vi "ButtonEvents.vi"(11 "UiDefinition":T1) -> ()   [LabVIEW 2020]
uses:
  UIReferences.ctl
  C:/Users/User/Desktop/Automation/NextVersion2/LabviewDXFViewer/bin/Release/LabviewDXFViewer.exe
  LabviewDXFViewer/bin/Release/LabviewDXFViewer.exe
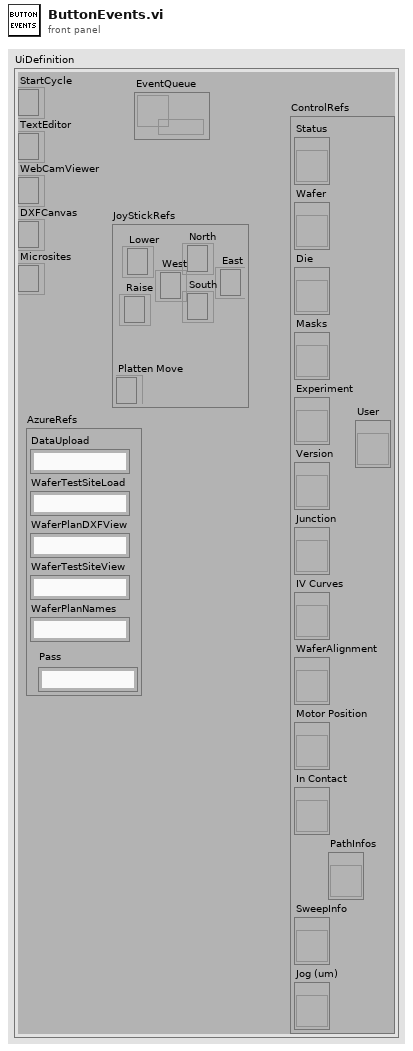
[diagram p1: front panel]
types:
  T1 = typedef "UIReferences.ctl" = cluster{"StartCycle":refnum<k24>, "TextEditor":refnum<k24>, "WebCamViewer":refnum<k24>, "DXFCanvas":refnum<k24>, "Microsites":refnum<k24>, "JoyStickRefs":cluster{"North":refnum<k24>, "Lower":refnum<k24>, "Raise":refnum<k24>, "Platten Move":refnum<k24>, "West":refnum<k24>, "East":refnum<k24>, "South":refnum<k24>}, "AzureRefs":cluster{"DataUpload":string, "WaferTestSiteLoad":string, "WaferPlanDXFView":string, "WaferTestSiteView":string, "WaferPlanNames":string, "Pass":string}, "ControlRefs":cluster{"Status":refnum<vi>, "Wafer":refnum<vi>, "Die":refnum<vi>, "Masks":refnum<vi>, "Experiment":refnum<vi>, "Version":refnum<vi>, "Junction":refnum<vi>, "IV Curves":refnum<vi>, "WaferAlignment":refnum<vi>, "Motor Position":refnum<vi>, "In Contact":refnum<vi>, "SweepInfo":refnum<vi>, "Jog (um)":refnum<vi>, "PathInfos":refnum<vi>, "User":refnum<vi>}, "EventQueue":refnum<queue>}
  T2 = cluster{"North":refnum<k24>, "Lower":refnum<k24>, "Raise":refnum<k24>, "Platten Move":refnum<k24>, "West":refnum<k24>, "East":refnum<k24>, "South":refnum<k24>}
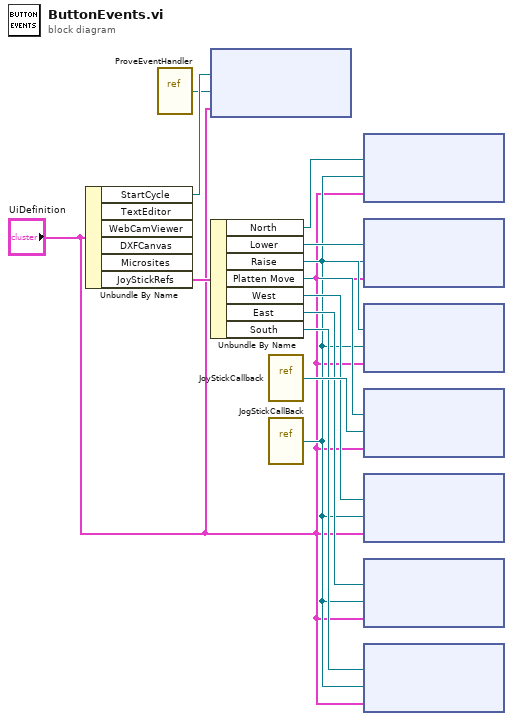
[diagram p0: block diagram]
diagram:
  n1 = Unbundle By Name("UiDefinition") -> ("StartCycle"=w12:refnum<k24>, "JoyStickRefs"=w13:T2)  [unwired: 4 out]
  n2 = vi-ref "ProveEventHandler.vi"() -> ("vi reference"=w11:refnum<vi>)
  n3 = node(w12, w11, "UiDefinition") -> ()  [unwired: 2 in, 2 out]
  n4 = Unbundle By Name(w13) -> ("North"=w4:refnum<k24>, "Lower"=w8:refnum<k24>, "Raise"=w7:refnum<k24>, "Platten Move"=w10:refnum<k24>, "West"=w6:refnum<k24>, "East"=w5:refnum<k24>, "South"=w3:refnum<k24>)
  n5 = vi-ref "JoyStickCallback.vi"() -> ("vi reference"=w9:refnum<vi>)
  n6 = vi-ref "JogStickCallBack.vi"() -> ("vi reference"=w2:refnum<vi>)
  n7 = node(w4, w2, "UiDefinition") -> ()  [unwired: 2 in, 2 out]
  n8 = node(w8, w2, "UiDefinition") -> ()  [unwired: 2 in, 2 out]
  n9 = node(w7, w2, "UiDefinition") -> ()  [unwired: 2 in, 2 out]
  n10 = node(w10, w9, "UiDefinition") -> ()  [unwired: 2 in, 2 out]
  n11 = node(w6, w2, "UiDefinition") -> ()  [unwired: 2 in, 2 out]
  n12 = node(w5, w2, "UiDefinition") -> ()  [unwired: 2 in, 2 out]
  n13 = node(w3, w2, "UiDefinition") -> ()  [unwired: 2 in, 2 out]
